vi "Resideo Get All Vesta Data.vi"(8 "error in (no error)":errorcluster, 11 "Modbus Master in":refnum<class "Modbus Master.lvclass">) -> (0 "error out":errorcluster, 1 "Vesta Is Working":bool, 2 "Vesta Data Output":T1, 3 "Modbus Master out":refnum<class "Modbus Master.lvclass">)   [LabVIEW 2023]
uses:
  Type Definitions/Vesta Info.ctl
  <vilib>/NI/Modbus Library/API/Master/Modbus Master.lvclass
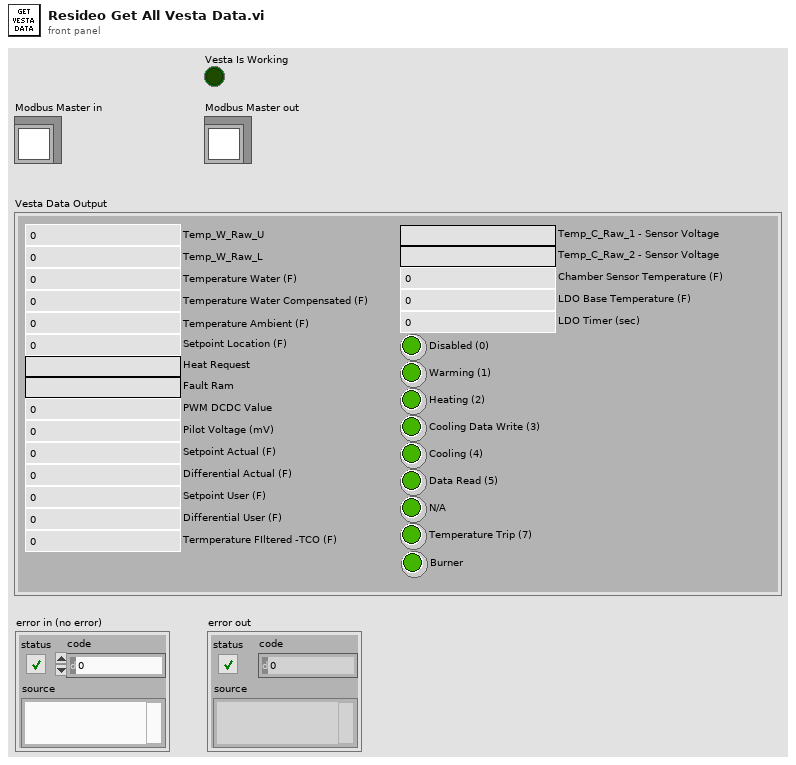
[diagram p1: front panel]
types:
  T1 = typedef "Vesta Info.ctl" = cluster{"Temp_W_Raw_U":u16, "Temp_W_Raw_L":u16, "Temperature Water (F)":dbl, "Temperature Water Compensated (F)":dbl, "Temperature Ambient (F)":dbl, "Setpoint Location (F)":dbl, "Heat Request":string, "Fault Ram":string, "PWM DCDC Value":u16, "Pilot Voltage (mV)":dbl, "Setpoint Actual (F)":dbl, "Differential Actual (F)":dbl, "Setpoint User (F)":dbl, "Differential User (F)":dbl, "Termperature FIltered -TCO (F)":dbl, "Temp_C_Raw_1 - Sensor Voltage":string, "Temp_C_Raw_2 - Sensor Voltage":string, "Chamber Sensor Temperature (F)":dbl, "LDO Base Temperature (F)":dbl, "LDO Timer (sec)":i16, "Disabled (0)":bool, "Warming (1)":bool, "Heating (2)":bool, "Cooling Data Write (3)":bool, "Cooling (4)":bool, "Data Read (5)":bool, "N/A":bool, "Temperature Trip (7)":bool, "Burner":bool}
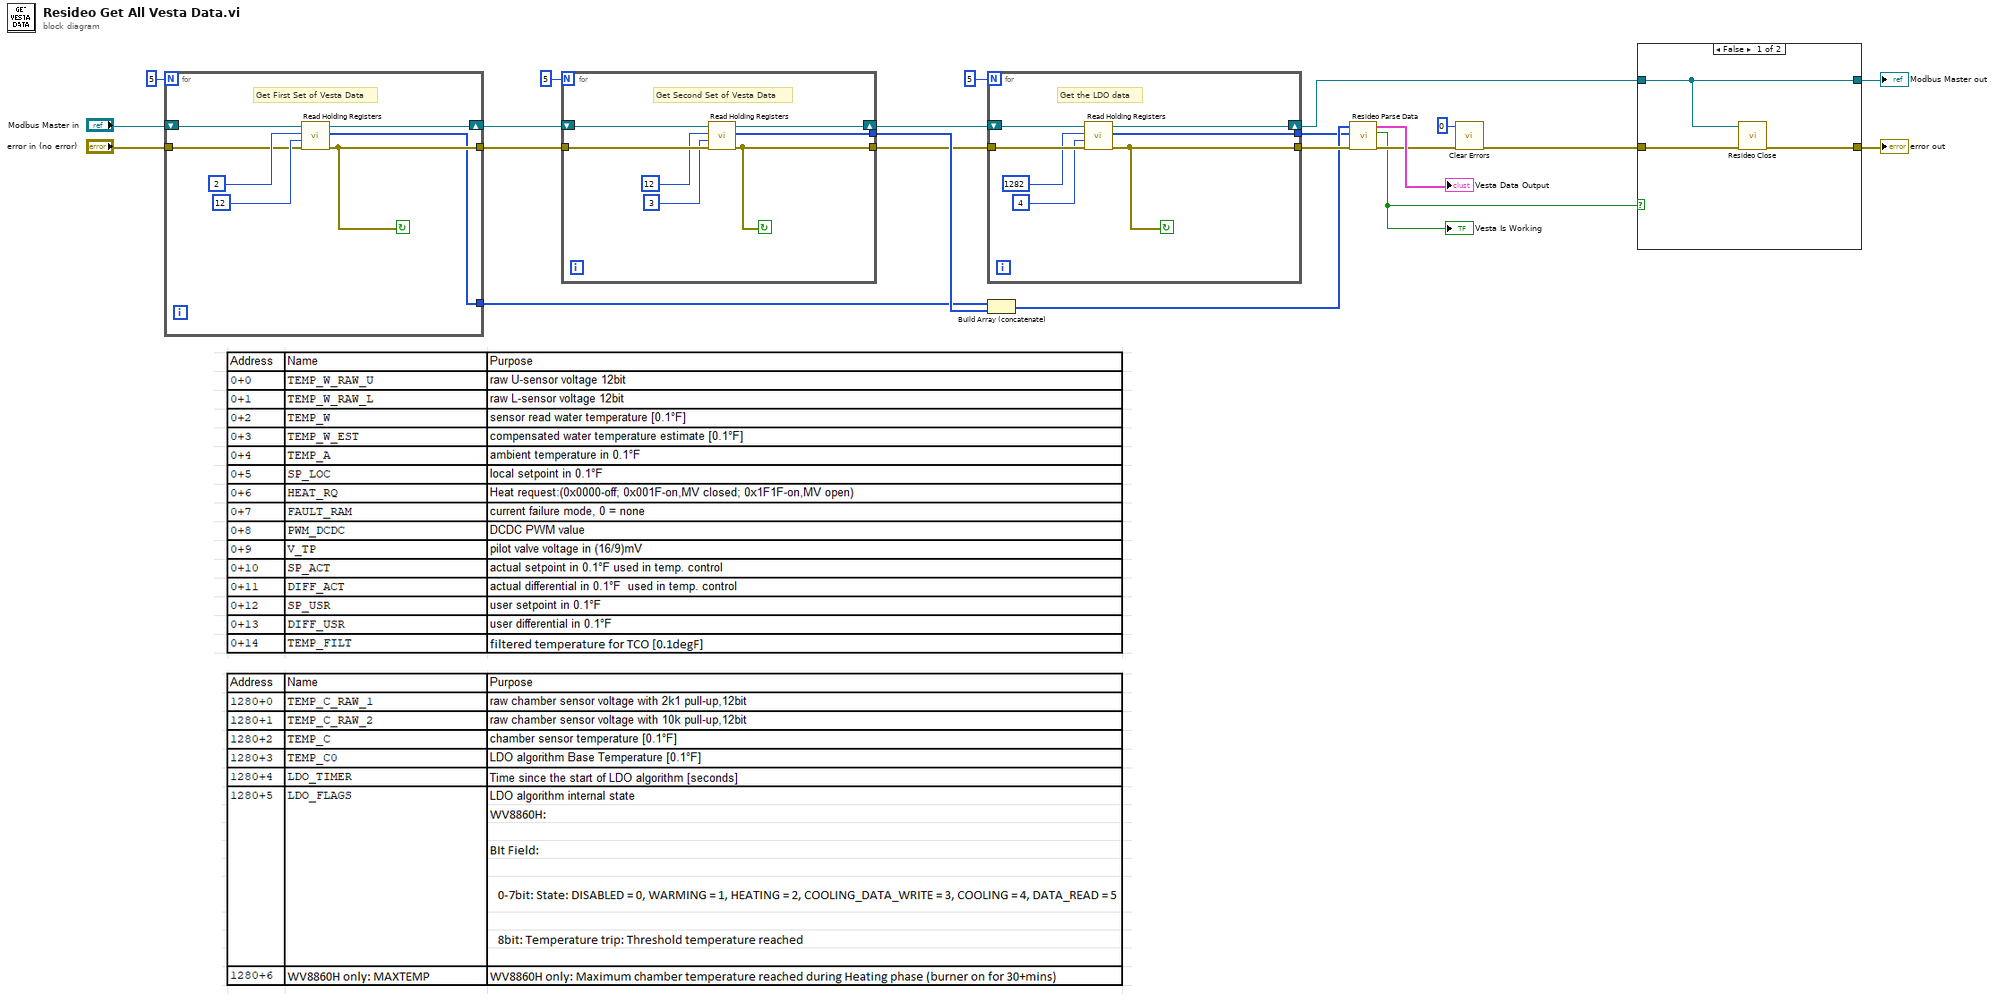
[diagram p0: block diagram]
diagram:
  n1 = for {
    N: 5 -> [_]
    tunnel: [w23] -> w18
    shift-right: [w29] -> w14
    shift-left: "Modbus Master in" -> [w25]
    tunnel: "error in (no error)" -> [w26]
    tunnel: [w24] -> w15
    stop <- w24 continue-if-true
    # "Get First Set of Vesta Data"
    n2 = call-dynamic "Read Holding Registers.vi"("error in"=w26, "number of inputs"=12 ("Register"), "starting address"=u16 2, "Modbus master in"=w25) -> ("error out"=w24:errorcluster, "register values"=w23:u16[], "Modbus master out"=w29:refnum<class "Modbus Master.lvclass">)  [unwired: 5 in]
  }
  n3 = for {
    N: 5 -> [_]
    tunnel: [w30] -> w19
    shift-right: [w36] -> w16
    shift-left: w14 -> [w34]
    tunnel: w15 -> [w35]
    tunnel: [w31] -> w17
    stop <- w31 continue-if-true
    # "Get Second Set of Vesta Data"
    n4 = call-dynamic "Read Holding Registers.vi"("error in"=w35, "number of inputs"=3 ("Register"), "starting address"=u16 12, "Modbus master in"=w34) -> ("error out"=w31:errorcluster, "register values"=w30:u16[], "Modbus master out"=w36:refnum<class "Modbus Master.lvclass">)  [unwired: 5 in]
  }
  n5 = for {
    N: 5 -> [_]
    tunnel: [w37] -> w13
    shift-right: [w41] -> w4
    shift-left: w16 -> [w42]
    tunnel: w17 -> [w43]
    tunnel: [w38] -> w21
    stop <- w38 continue-if-true
    # "Get the LDO data"
    n6 = call-dynamic "Read Holding Registers.vi"("error in"=w43, "number of inputs"=4 ("Register"), "starting address"=u16 1282, "Modbus master in"=w42) -> ("error out"=w38:errorcluster, "register values"=w37:u16[], "Modbus master out"=w41:refnum<class "Modbus Master.lvclass">)  [unwired: 5 in]
  }
  n7 = Build Array (concatenate)(w18, w19) -> (w20:u16[])
  n8 = call "Resideo Parse Data.vi"("error in (no error)"=w21, "LDO Data"=w13, "Vesta Data 1"=w20) -> ("error out"=w10:errorcluster, "Vesta Is Working"=w5:bool, "Vesta Data Output"=→"Vesta Data Output":T1)  [unwired: 6 in]
  "Vesta Is Working" <- w5
  n9 = call <vilib>:"Clear Errors.vi"("error in (no error)"=w10, "specific error code to clear (0: all)"=0) -> ("error out"=w2:errorcluster)  [unwired: 4 in, 1 out]
  n10 = case shown="False" w5 {
    tunnel: w4 -> [w46 w48]
    tunnel: [w46 w48] -> w3
    tunnel: w2 -> [w45 w47]
    tunnel: [w44 w47] -> w1
    frame False {
      n11 = call "Resideo Close.vi"("error in (no error)"=w45, "Modbus Master in"=w46) -> ("error out"=w44:errorcluster)  [unwired: 9 in]
    }
    frame True {
    }
  }
  "error out" <- w1
  "Modbus Master out" <- w3
